vi "Config_Populate.vi"(8 "error in (no error)":errorcluster, 11 "Config Ref In":T1) -> (0 "error out":errorcluster, 3 "refnum out":T1)   [LabVIEW 2021]
uses:
  <vilib>/Utility/config.llb/Config Data RefNum.ctl
  Config_Cluster.ctl
  <vilib>/Utility/config.llb/Write Key (Path).vi
  <vilib>/Utility/config.llb/Write Key (String).vi
  <vilib>/Utility/config.llb/Write Key (I32).vi
  <vilib>/Utility/config.llb/NI_LVConfig.lvlib
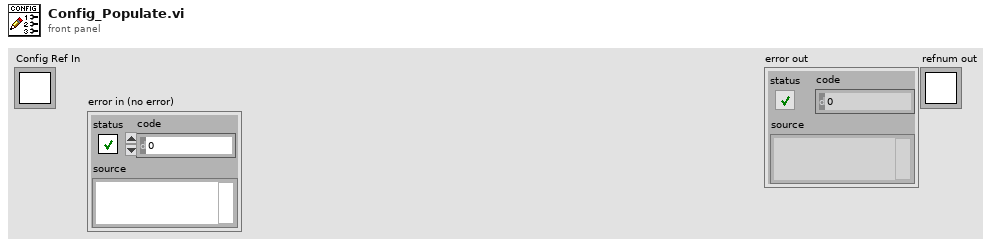
[diagram p1: front panel]
types:
  T1 = typedef "NI_LVConfig.lvlib/Config Data RefNum.ctl" = refnum<k1>
  T2 = typedef "Config_Cluster.ctl" = cluster{"General":cluster{"Config.ini":path, "Default Logging Path":path}, "Hardware":cluster{"LCR VISA COM":refnum<visa-resource-name>, "Measure Rate (1/s)":i32, "Reset on Load?":bool, "Measure Profile":path}, "HM8118 Current Profile":cluster{"Bias Profile":cluster{" Bias Source (OFF)":u8, " Bias Type (Voltage)":u8, "Bias Level (0)":dbl}, "Measurement Profile":cluster{"Operation Mode (0: Auto)":u16, "Circuit Type (2: Auto)":u16, "Manual Range (1:Range 1 and 25 Ohms)":u8, "Auto Range (T: Enable)":bool}, "Signal Profile":cluster{"Frequency (1kHz)":dbl, "Measuring Voltage (1V)":dbl}, "Integration Profile":cluster{"Averaging (0: Off)":u16, "Averaging Number (2)":i32, "Time (100ms)":i32, "Rate (0: Fast)":u16}, "Trigger Profile":cluster{"Trigger Mode (0: Continuous)":u16}}, "HM8118 New Profile":cluster{"Bias Profile":cluster{" Bias Source (OFF)":u8, " Bias Type (Voltage)":u8, "Bias Level (0)":dbl}, "Measurement Profile":cluster{"Operation Mode (0: Auto)":u16, "Circuit Type (2: Auto)":u16, "Manual Range (1:Range 1 and 25 Ohms)":u8, "Auto Range (T: Enable)":bool}, "Signal Profile":cluster{"Frequency (1kHz)":dbl, "Measuring Voltage (1V)":dbl}, "Integration Profile":cluster{"Averaging (0: Off)":u16, "Averaging Number (2)":i32, "Time (100ms)":i32, "Rate (0: Fast)":u16}, "Trigger Profile":cluster{"Trigger Mode (0: Continuous)":u16}}}
  T3 = cluster{"Config.ini":path, "Default Logging Path":path}
  T4 = cluster{"LCR VISA COM":refnum<visa-resource-name>, "Measure Rate (1/s)":i32, "Reset on Load?":bool, "Measure Profile":path}
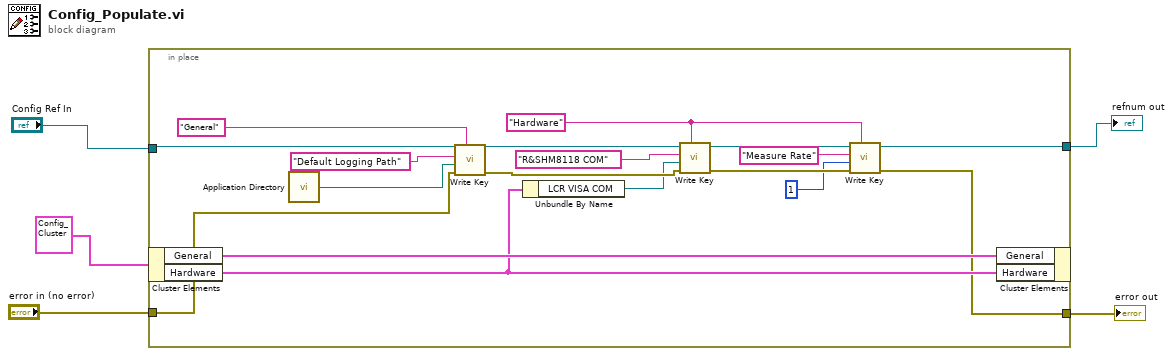
[diagram p0: block diagram]
diagram:
  n1 = in-place {
    in-place-border: "Config Ref In" -> [w23]
    in-place-border: "error in (no error)" -> [w22]
    in-place-border: [w9] -> w2
    in-place-border: [w8] -> w1
    w12 = "Hardware" ("section")
    n2 = in-place-cluster #1(T2 {"General"={"Config.ini"=path "", "Default Logging Path"=path ""}, "Hardware"={"LCR VISA COM"="COM1", "Measure Rate (1/s)"=1, "Reset on Load?"=FALSE, "Measure Profile"=path ""}, "HM8118 Current Profile"={"Bias Profile"={" Bias Source (OFF)"=0, " Bias Type (Voltage)"=0, "Bias Level (0)"=0.0}, "Measurement Profile"={"Operation Mode (0: Auto)"=0, "Circuit Type (2: Auto)"=2, "Manual Range (1:Range 1 and 25 Ohms)"=1, "Auto Range (T: Enable)"=TRUE}, "Signal Profile"={"Frequency (1kHz)"=1000.0, "Measuring Voltage (1V)"=1.0}, "Integration Profile"={"Averaging (0: Off)"=0, "Averaging Number (2)"=2, "Time (100ms)"=100, "Rate (0: Fast)"=0}, "Trigger Profile"={"Trigger Mode (0: Continuous)"=0}}, "HM8118 New Profile"={"Bias Profile"={" Bias Source (OFF)"=0, " Bias Type (Voltage)"=0, "Bias Level (0)"=0.0}, "Measurement Profile"={"Operation Mode (0: Auto)"=0, "Circuit Type (2: Auto)"=2, "Manual Range (1:Range 1 and 25 Ohms)"=1, "Auto Range (T: Enable)"=TRUE}, "Signal Profile"={"Frequency (1kHz)"=1000.0, "Measuring Voltage (1V)"=1.0}, "Integration Profile"={"Averaging (0: Off)"=0, "Averaging Number (2)"=2, "Time (100ms)"=100, "Rate (0: Fast)"=0}, "Trigger Profile"={"Trigger Mode (0: Continuous)"=0}}} ("Configuration Cluster")) -> ("General"=w19:T3, "Hardware"=w18:T4)
    n3 = call <vilib>:"Application Directory.vi"() -> ("Application Directory"=w7:path)
    n4 = call-poly <vilib>:"Write Key.vi"("section"="General", "error in (no error)"=w22, "value"=w7, "key"="Default Logging Path", "refnum"=w23) -> ("error out"=w17:errorcluster, "refnum out"=w20:T1)  [unwired: 4 in, 1 out]
    n5 = Unbundle By Name(w18) -> ("LCR VISA COM"=w15:refnum<visa-resource-name>)
    n6 = call-poly <vilib>:"Write Key.vi"("section"=w12, "error in (no error)"=w17, "value"=w15, "key"="R&SHM8118 COM", "refnum"=w20) -> ("error out"=w11:errorcluster, "refnum out"=w13:T1)  [unwired: 4 in, 1 out]
    n7 = call-poly <vilib>:"Write Key.vi"("section"=w12, "error in (no error)"=w11, "value"=1 ("Measure Rate (1/s)"), "key"="Measure Rate", "refnum"=w13) -> ("error out"=w9:errorcluster, "refnum out"=w8:T1)  [unwired: 4 in, 1 out]
    n8 = in-place-cluster #1("General"=w19, "Hardware"=w18) -> ()  [unwired: 1 out]
  }
  "error out" <- w2
  "refnum out" <- w1
